vi "ex_WriteDataTDM.vi"(0 "file path":path, 1 "first call":bool, 2 "Lock file":bool, 3 "Signals":waveform(dbl)[](array[waveform]), 4 "overwrite_mode_multi":T8(ring)=enum."overwrite & backup", 5 "overwrite_mode":T9(ring)=enum."overwrite & backup", 7 "error in (no error)":errorcluster, 8 "file dialog?":bool, 9 "Description":string, 12 "multi_file":bool, 13 "Comment":string, 14 "new file?":bool, 15 "Simulate Non-First Call":bool, 16 "file params":T6={"delimiter"="\t", "origin time"=timestamp(0 s since 1904-01-01), "Flags"={"include col headings?"=TRUE, "x_columns"=0, "col headings always?"=TRUE, "time preference"=0, "hide col headings"=FALSE}, "Decimal Separator"=""} {"Flags"."time preference" items=["Absolute", "Relative"]; "Flags"."x_columns" items=["None", "One", "Multiple"]; "origin time" format="%<%X\n%x>T"}, 23 "append info":T1, 25 "DAQmx Task":T2) -> (17 "operator cancelled?":bool, 20 "file path out":path, 21 "bytes written":i32, 24 "append info out":T1, 27 "error out":errorcluster)   [LabVIEW 2020]
uses:
  <vilib>/express/express output/ExFileWriteBlock.llb/ex_WriteFileParams.ctl
  <vilib>/express/express input/ExFileReadBlock.llb/ex_ReadFileParams.ctl
  <vilib>/express/express shared/ex_EditUserDefinedProperties/ex_userdefproperties.ctl
  <vilib>/express/express shared/ExFile.llb/ex_userDefProperty.ctl
  <vilib>/express/express shared/ex_EditUserDefinedProperties/usiDataType.ctl
  <vilib>/express/express shared/ExFile.llb/ex_propertySource.ctl
  <vilib>/Platform/express/TDMExpress.llb/ex_appendInfoTDM.ctl
  <vilib>/Platform/storage/Storage.llb/__closeStorageFromObject.vi
panel:
  in  "automatic headers":bool
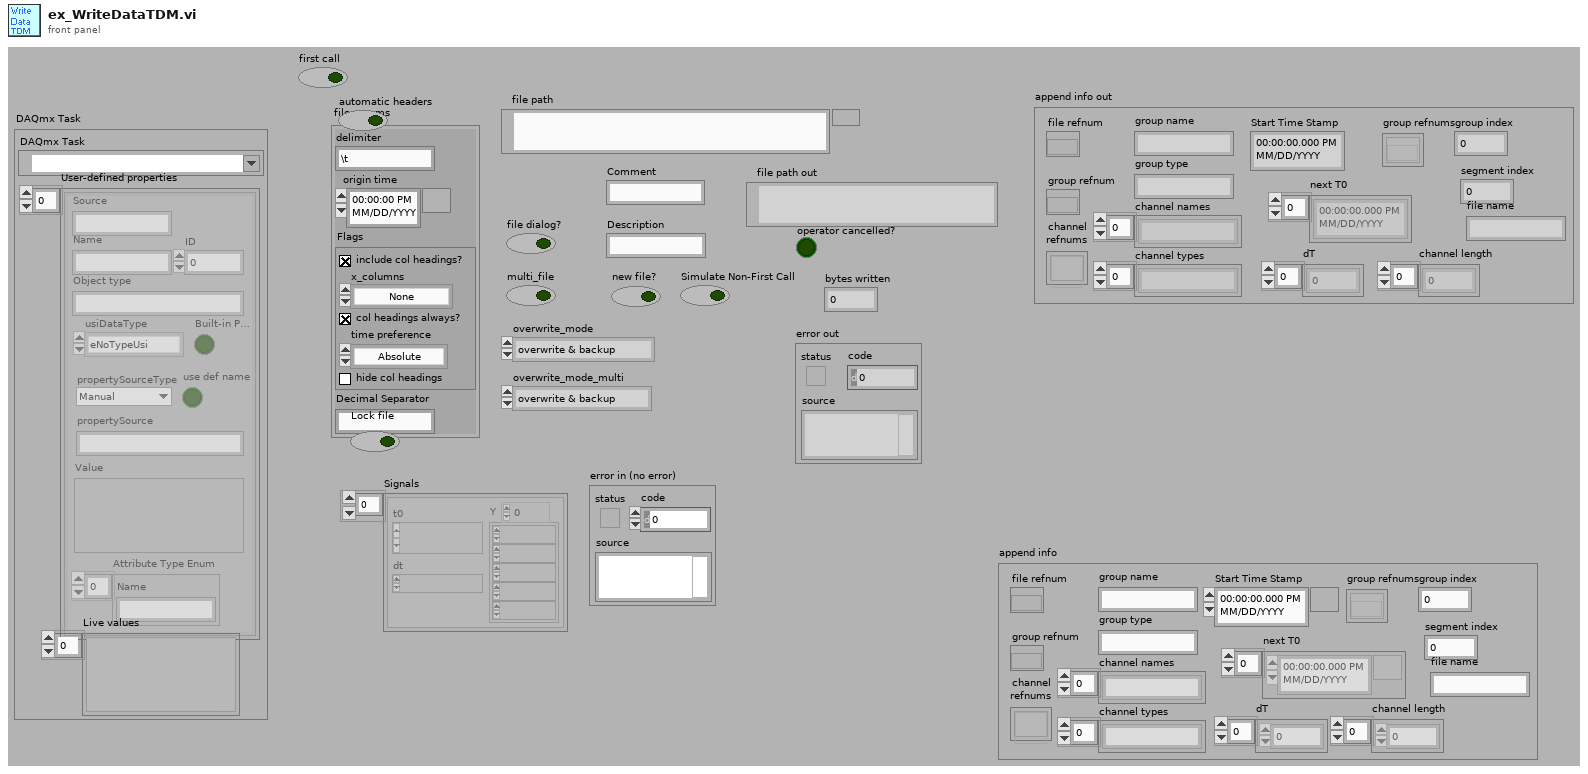
[diagram p1: front panel]
types:
  T1 = typedef "ex_appendInfoTDM.ctl" = cluster{"channel\nrefnums":refnum<k20>[], "channel names":string[], "channel types":string[], "file refnum":refnum<k20>, "group refnum":refnum<k20>, "group name":string, "group type":string, "next T0":timestamp[], "dT":dbl[], "Start Time Stamp":timestamp, "channel length":u32[], "group index":u32, "group refnums":refnum<k20>[], "file name":string, "segment index":u32}
  T2 = typedef "ex_userdefproperties.ctl" = cluster{"DAQmx Task":refnum<k21>, "User-defined properties":T3[], "Live values":variant[]}
  T3 = typedef "ex_userDefProperty.ctl" = cluster{"Name":string, "Object type":string, "usiDataType":T4, "propertySourceType":T5, "propertySource":string, "Value":variant, "ID":i32, "use def name":bool, "Source":string, "Built-in Prop":bool, "Attribute Type Enum":string[]}
  T4 = typedef "usiDataType.ctl" = enum16{"eNoTypeUsi", "eInt8Usi", "eInt16Usi", "eInt32Usi", "eInt64Usi", "eUInt8Usi", "eUInt16Usi", "eUInt32Usi", "eUInt64Usi", "eFloat32Usi", "eFloat64Usi", "- 0", "- 1", "- 2", "- 3", "- 4", "- 5", "- 6", "- 7", "- 8", "- 9", "eString8Usi", "eString16Usi", "eStringUsi", "eEnumUsi", "- 10", "- 11", "- 12", "- 13", "- 14", "eTimeUsi", "- 15", "- 16", "- 17", "- 18", "- 19", "- 20", "- 21", "- 22", "- 23", "eInstanceUsi", "eStoreUsi"}
  T5 = typedef "ex_propertySource.ctl" = enum16{"Manual", "System", "DAQmx Channel", "Terminal", "Ignore"}
  T6 = typedef "ex_WriteFileParams.ctl" = cluster{"delimiter":string, "origin time":timestamp, "Flags":T7, "Decimal Separator":string}
  T7 = typedef "ex_ReadFileParams.ctl" = cluster{"include col headings?":bool, "x_columns":u16, "col headings always?":bool, "time preference":u16, "hide col headings":bool}
  T8 = enum16{"overwrite", "overwrite & backup", "next avail"}
  T9 = enum16{"overwrite", "overwrite & backup", "append", "next avail"}
  T10 = cluster{"Start Timestamp":timestamp, "Timestamp":timestamp, "Relative Time?":bool, "X Dimension":string, "Signal Name":string, "Y Units":string, "X0":timestamp, "dX":dbl, "nPoints":i32}[]
  T11 = typedef "ex_WaveformAttribsPlus.ctl" = cluster{"Start Timestamp":timestamp, "Timestamp":timestamp, "Relative Time?":bool, "X Dimension":string, "Signal Name":string, "Y Units":string, "X0":timestamp, "dX":dbl, "nPoints":i32}
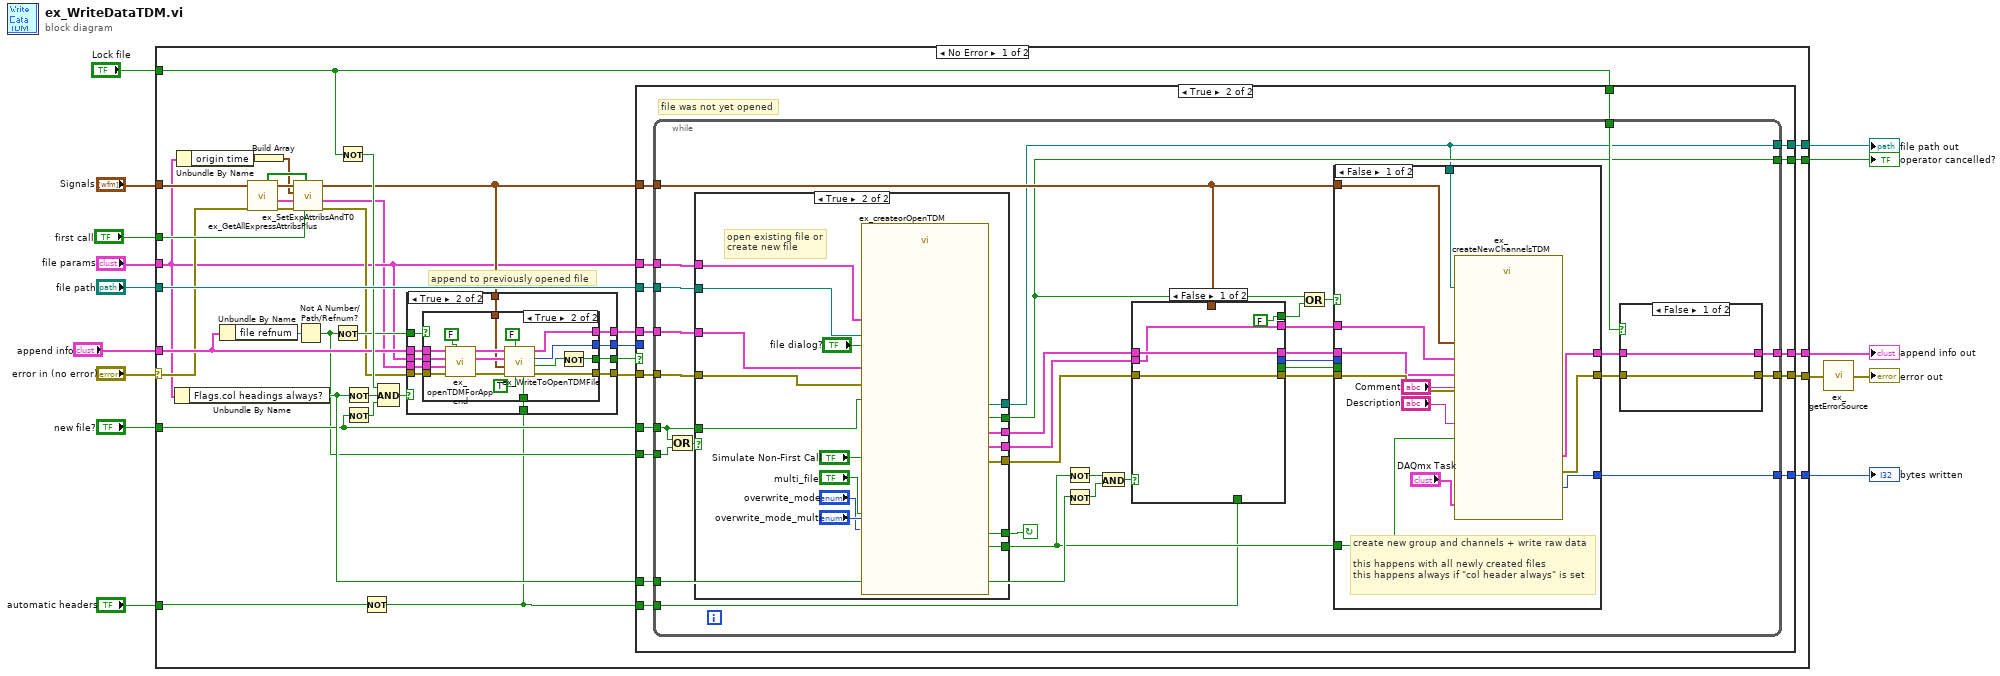
[diagram p0: block diagram]
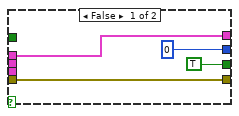
[diagram p2: hidden frame]
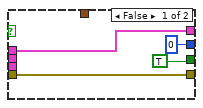
[diagram p3: hidden frame]
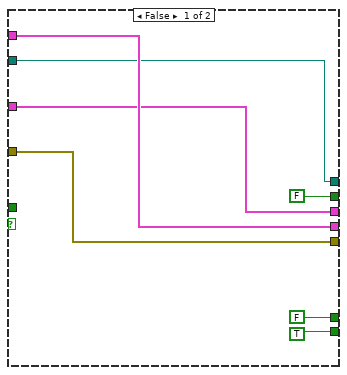
[diagram p5: hidden frame]
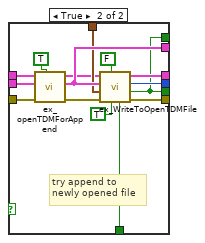
[diagram p6: hidden frame]
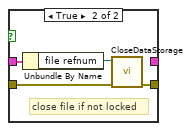
[diagram p7: hidden frame]
diagram:
  n1 = case shown="No Error" "error in (no error)" {
    selector: "error in (no error)" -> [w21 w206]
    tunnel: [w51 w206] -> w15
    tunnel: "Signals" -> [w24 _]
    tunnel: "new file?" -> [w41 _]
    tunnel: "file params" -> [w18 _]
    tunnel: [w47 w205] -> w1
    tunnel: "file path" -> [w45 w204]
    tunnel: "append info" -> [w37 w205]
    tunnel: "Lock file" -> [w44 _]
    tunnel: [w33 w204] -> w8
    tunnel: [w32 _] -> w7
    tunnel: [w31 _] -> w6
    tunnel: "automatic headers" -> [w30 _]
    tunnel: "first call" -> [w22 _]
    frame No Error {
      # "append to previously opened file"
      n2 = Unbundle By Name(w18) -> ("Flags.col headings always?"=w42:bool)
      n3 = Unbundle By Name(w18) -> ("origin time"=w19:timestamp)
      n4 = Unbundle By Name(w37) -> ("file refnum"=w38:refnum<k20>)
      n5 = call <vilib>:"ex_GetAllExpressAttribsPlus.vi"("error in"=w21, "Signals in"=w24) -> ("error out"=w28:errorcluster, "All Express Wave Attributes Plus"=w27:T10, "Signals out"=w26:waveform(dbl)[], "Time Attribs Not Found"=w25:bool[])  [unwired: 6 out]
      n6 = Build Array(w19) -> (w17:timestamp[])
      n7 = call <vilib>:"ex_SetExpAttribsAndT0.vi"("Latch Origin TS? (T)"=w22, "Set? (T if empty)"=w25, "error in (no error)"=w28, "Express Attributes Plus in"=w27, "Origin Timestamps"=w17, "Signals"=w26) -> ("error out"=w20:errorcluster, "Express Wave Attributes Plus out"=w16:T11[], "Signals With Attributes"=w23:waveform(dbl)[])  [unwired: 3 out]
      n8 = Not A Number/Path/Refnum?(number/path/refnum=w38) -> (NaN/Path/Refnum?=w34:bool)
      n9 = Not(x=w34) -> (.not. x?=w36:bool)
      n10 = Not(x=w44) -> (.not. x?=w40:bool)
      n11 = Not(x=w42) -> (.not. x?=w39:bool)
      n12 = Not(x=w41) -> (.not. x?=w35:bool)
      n13 = Not(x=w30) -> (.not. x?=w29:bool)
      n14 = Compound Arithmetic op=AND(w40, w39, w35) -> (w43:bool)
      n15 = case shown="True" w43 {
        tunnel: w20 -> [w55 w66]
        tunnel: [w55 w65] -> w50
        tunnel: w18 -> [_ w62]
        tunnel: [TRUE w61] -> w46
        tunnel: [0 w64] -> w49
        tunnel: [w54 w63] -> w48
        tunnel: w37 -> [w54 w60]
        tunnel: w36 -> [_ w59]
        tunnel: w23 -> [_ w58]
        tunnel: w29 -> [_ w57]
        tunnel: w16 -> [_ w56]
        frame False {
        }
        frame True {
          n16 = case shown="True" w59 {
            tunnel: w66 -> [w69 w83]
            tunnel: [w69 w87] -> w65
            tunnel: [0 ("bytes written") w86] -> w64
            tunnel: [w70 w85] -> w63
            tunnel: w62 -> [_ w82]
            tunnel: [TRUE w75] -> w61
            tunnel: w60 -> [w70 w81]
            tunnel: w58 -> [_ w77]
            tunnel: w57 -> [_ w76]
            tunnel: w56 -> [_ w72]
            frame False {
            }
            frame True {
              n17 = call <vilib>:"ex_openTDMForAppend.vi"("always read cache"=FALSE, "error in (no error)"=w83, "Express Wave Attributes Plus in"=w72, "file params"=w82, "append info in"=w81) -> ("error out"=w80:errorcluster, "file params out"=w79:T6, "append info out"=w78:T1)  [unwired: 4 out]
              n18 = call <vilib>:"ex_WriteToOpenTDMFile.vi"("error if check fails"=w76, "check time attributes"=TRUE, "write ddt attr"=FALSE, "error in (no error)"=w80, "Signals"=w77, "file params"=w79, "append info in"=w78) -> ("error out"=w87:errorcluster, "open file was used"=w74:bool, "bytes written"=w86:i32, "append info out"=w85:T1)  [unwired: 1 in]
              n19 = Not(x=w74) -> (.not. x?=w75:bool)
            }
          }
        }
      }
      n20 = case shown="True" w46 {
        tunnel: [w89 w106] -> w51
        tunnel: [w91 w105] -> w31
        tunnel: w41 -> [_ w104]
        tunnel: w50 -> [w89 w103]
        tunnel: w18 -> [_ w102]
        tunnel: w49 -> [w91 _]
        tunnel: w48 -> [w90 w98]
        tunnel: [w90 w101] -> w47
        tunnel: w45 -> [w88 w100]
        tunnel: w44 -> [_ w99]
        tunnel: w23 -> [_ w97]
        tunnel: w42 -> [_ w96]
        tunnel: w34 -> [_ w95]
        tunnel: [w88 w94] -> w33
        tunnel: [_ w93] -> w32
        tunnel: w29 -> [_ w92]
        frame False {
        }
        frame True {
          # "file was not yet opened"
          n21 = while {
            tunnel: w103 -> [w139]
            tunnel: w104 -> [w113]
            tunnel: w100 -> [w138]
            tunnel: [w107] -> w94
            tunnel: [w120] -> w93
            tunnel: [w134] -> w106
            tunnel: [w137] -> w105
            tunnel: w102 -> [w136]
            tunnel: [w132] -> w101
            tunnel: w99 -> [w133]
            tunnel: w98 -> [w123]
            tunnel: w97 -> [w124]
            tunnel: w96 -> [w117]
            tunnel: w95 -> [w118]
            tunnel: w92 -> [w108]
            stop <- w135 continue-if-true
            n22 = Or(x=w113, y=w118) -> (x .or. y?=w119:bool)
            n23 = case shown="True" w119 {
              tunnel: w139 -> [w144 w163]
              tunnel: w138 -> [w143 w162]
              tunnel: w136 -> [w146 w160]
              tunnel: [FALSE ("keep loop going") w155] -> w135
              tunnel: [w143 w154] -> w107
              tunnel: [w144 w153] -> w130
              tunnel: [w146 w152] -> w128
              tunnel: w113 -> [_ w151]
              tunnel: w123 -> [w145 w150]
              tunnel: [w145 w149] -> w122
              tunnel: [FALSE ("dialog was cancelled") w148] -> w120
              tunnel: [TRUE ("keep loop going") w147] -> w111
              frame False {
              }
              frame True {
                # "open existing file or\ncreate new file"
                n24 = call <vilib>:"ex_createorOpenTDM.vi"("file path in"=w162, "overwrite_mode_multi"="overwrite_mode_multi", "overwrite_mode"="overwrite_mode", "append info in"=w150, "file dialog?"="file dialog?", "error in (no error)"=w163, "file params"=w160, "multi_file"="multi_file", "new file?"=w151, "Simulate Non-First Call"="Simulate Non-First Call") -> ("new file was created"=w147:bool, "file path out"=w154:path, "dialog was cancelled"=w148:bool, "keep loop going"=w155:bool, "append info out"=w149:T1, "file params out"=w152:T6, "error out"=w153:errorcluster)  [unwired: 3 out]
              }
            }
            n25 = Not(x=w111) -> (.not. x?=w112:bool)
            n26 = Not(x=w117) -> (.not. x?=w116:bool)
            n27 = And(x=w112, y=w116) -> (x .and. y?=w115:bool)
            n28 = case shown="False" w115 {
              tunnel: w130 -> [w167 w182]
              tunnel: [w167 w181] -> w129
              tunnel: w128 -> [w165 w179]
              tunnel: [w165 w178] -> w127
              tunnel: [w166 w177] -> w126
              tunnel: [_ w176] -> w125
              tunnel: w124 -> [_ w175]
              tunnel: w122 -> [w166 w174]
              tunnel: [_ w171] -> w121
              tunnel: [FALSE w171] -> w114
              tunnel: w108 -> [_ w170]
              frame False {
              }
              frame True {
                # "try append to \nnewly opened file"
                n29 = call <vilib>:"ex_openTDMForAppend.vi"("always read cache"=TRUE, "error in (no error)"=w182, "file params"=w179, "append info in"=w174) -> ("error out"=w180:errorcluster, "file params out"=w178:T6, "append info out"=w173:T1)  [unwired: 1 in, 4 out]
                n30 = call <vilib>:"ex_WriteToOpenTDMFile.vi"("error if check fails"=w170, "check time attributes"=TRUE ("error if check fails"), "write ddt attr"=FALSE, "error in (no error)"=w180, "Signals"=w175, "file params"=w178, "append info in"=w173) -> ("error out"=w181:errorcluster, "open file was used"=w171:bool, "bytes written"=w176:i32, "append info out"=w177:T1)  [unwired: 1 in]
              }
            }
            n31 = Or(x=w120, y=w114) -> (x .or. y?=w131:bool)
            n32 = case shown="False" w131 {
              tunnel: w127 -> [w195 _]
              tunnel: [w197 w203] -> w109
              tunnel: w129 -> [w200 w203]
              tunnel: [w199 w202] -> w137
              tunnel: [w196 w201] -> w110
              tunnel: w121 -> [_ _]
              tunnel: w126 -> [w198 w201]
              tunnel: w125 -> [_ w202]
              tunnel: w124 -> [w194 _]
              tunnel: w111 -> [w193 _]
              tunnel: w107 -> [w189 _]
              frame False {
                # "create new group and channels + write raw data\n\nthis happens with all newly created files\nthis happens always if \"col header always\" is set"
                n33 = call <vilib>:"ex_createNewChannelsTDM.vi"("DAQmx Task"="DAQmx Task", "signals"=w194, "file params"=w195, "File path"=w189, "error in (no error)"=w200, "Comment"="Comment", "Description"="Description", "write file properties"=w193, "append info in"=w198) -> ("append info out"=w196:T1, "bytes written"=w199:i32, "error out"=w197:errorcluster)  [unwired: 4 out]
              }
              frame True {
              }
            }
            n34 = case shown="False" w133 {
              tunnel: w109 -> [w184 w188]
              tunnel: [w184 w187] -> w134
              tunnel: w110 -> [w183 w186]
              tunnel: [w183 _] -> w132
              frame False {
              }
              frame True {
                # "close file if not locked"
                n35 = Unbundle By Name(w186) -> ("file refnum"=w185:refnum<k20>)
                n36 = call-poly <vilib>:"CloseDataStorage.vi"("error in (no error)"=w188, "storage refnum"=w185) -> ("error out"=w187:errorcluster)  [unwired: 5 out]
              }
            }
          }
        }
      }
    }
    frame Error {
    }
  }
  "operator cancelled?" <- w7
  "file path out" <- w8
  "bytes written" <- w6
  "append info out" <- w1
  n37 = call <vilib>:"ex_getErrorSource.vi"("error in (no error)"=w15) -> ("error out"=→"error out":errorcluster)
